vi "DSF.Engine.Pool.ID.Destroy.vi"(8 "error in (no error)":errorcluster, 11 "ID Pool in":refnum<class "Pool ID.lvclass">) -> (0 "error out":errorcluster, 3 "ID Pool out":refnum<class "Pool ID.lvclass">)   [LabVIEW 2017, in "Data Sharing Framework Engine.lvlib" / "Pool ID.lvclass"]
uses:
  Pool ID.lvclass
  C:/github/data-sharing-framework/old/dsf core/Source/Engine/Classes/Thread Pool/Pool.lvclass
  Pool.lvclass
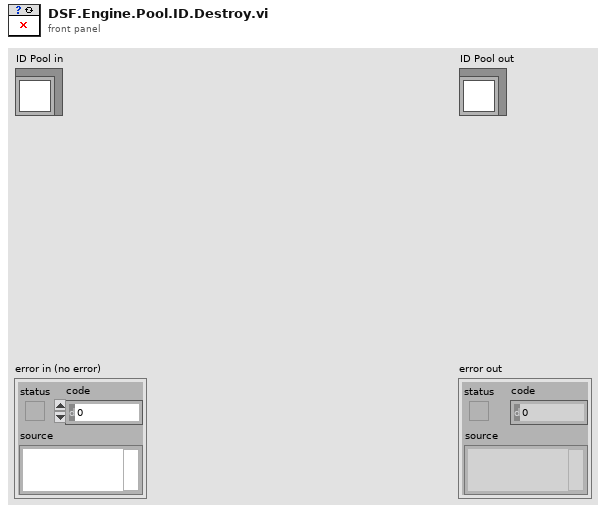
[diagram p1: front panel]
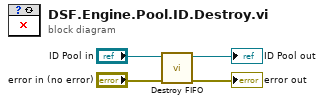
[diagram p0: block diagram]
diagram:
  n1 = call "Destroy FIFO.vi"("error in (no error)"="error in (no error)", "Pool in"="ID Pool in") -> ("error out"=→"error out":errorcluster, "Pool out"=→"ID Pool out":refnum<class "Pool ID.lvclass">)  [unwired: 8 in]
